vi "Read Serial Output Data Rate.vi"(0 "fpga interface in":refnum<k20>, 5 "serial output channels":string[](array[string]), 11 "error in (no error)":errorcluster) -> (4 "fpga interface out":refnum<k20>, 6 "serial output data rates (bps)":dbl[](array[numeric]), 15 "error out":errorcluster)   [LabVIEW 2023, in "GettingStarted_Common_148X_Host.lvlib"]
uses:
  GettingStarted_Common_148X_Host.lvlib
  <instrlib>/FlexRIO/API/Host/v1/NI FlexRIO/API/Get Property Reference - Fpga Small.vi
  <resource>/objmgr/niflexrioapiChannel.rc
  <instrlib>/FlexRIO/API/Host/v1/NI FlexRIO API v1.lvlib
  <resource>/objmgr/niflexrioapi.rc
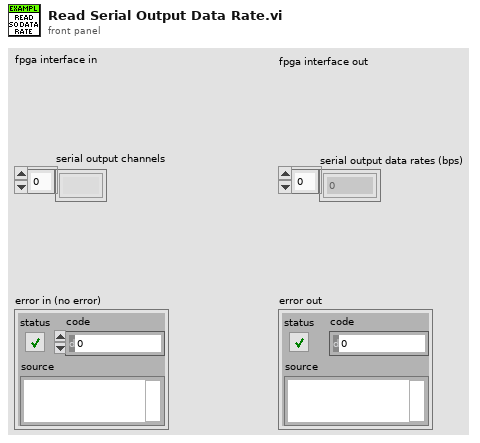
[diagram p1: front panel]
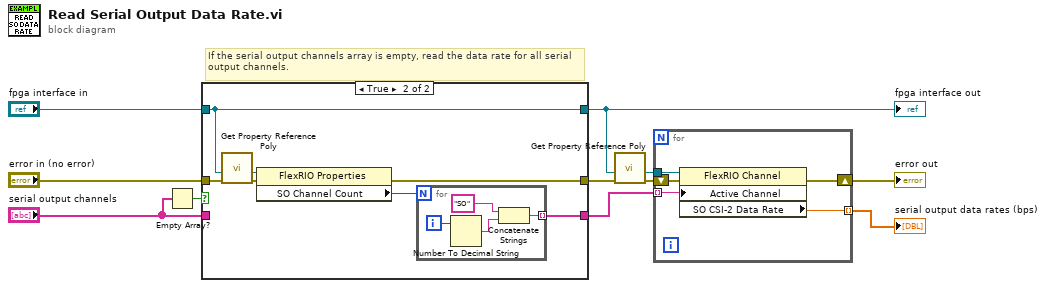
[diagram p0: block diagram]
diagram:
  # "If the serial output channels array is empty, read the data rate for all serial output channels."
  n1 = Empty Array?(array="serial output channels") -> (empty?=w5:bool)
  n2 = case shown="True" w5 {
    tunnel: "serial output channels" -> [w12 _]
    tunnel: "error in (no error)" -> [w13 w18]
    tunnel: [w12 w19] -> w1
    tunnel: "fpga interface in" -> [w14 w17]
    tunnel: [w14 w17] -> w3
    tunnel: [w13 w16] -> w2
    frame False {
    }
    frame True {
      n3 = call-poly <instrlib>:"Get Property Reference Poly.vi"("error in (no error)"=w18, "fpga interface in"=w17) -> ("error out"=w20:errorcluster, "property reference"=w21:refnum<k20>)  [unwired: 4 in, 1 out]
      n4 = property class="FlexRIO Properties"(reference=w21, error in=w20) -> (error out=w16:errorcluster, "SO Channel Count"=w15:i32)  [unwired: 1 out]
      n5 = for {
        N: w15 -> [_]
        tunnel: [w22] -> w19 mode=indexing
        i -> [w25]
        n6 = Number To Decimal String(number=w25) -> (decimal integer string=w24:string)  [unwired: 1 in]
        n7 = Concatenate Strings("SO", w24) -> (w22:string)
      }
    }
  }
  "fpga interface out" <- w3
  n8 = call-poly <instrlib>:"Get Property Reference Poly.vi"("error in (no error)"=w2, "fpga interface in"=w3) -> ("error out"=w11:errorcluster, "property reference"=w10:refnum<k20>)  [unwired: 4 in, 1 out]
  n9 = for {
    tunnel: w10 -> [w29]
    tunnel: w1 -> [w28] mode=indexing
    shift-right: [w27] -> w9
    shift-left: w11 -> [w30]
    tunnel: [w26] -> w8 mode=indexing
    n10 = property class="FlexRIO Channel"(reference=w29, error in=w30, "Active Channel"=w28) -> (error out=w27:errorcluster, "SO CSI-2 Data Rate"=w26:dbl)  [unwired: 1 out]
  }
  "error out" <- w9
  "serial output data rates (bps)" <- w8
